vi "ConfigureHW.vi"(8 "error in (no error)":errorcluster, 11 "BME_DG_Base in":refnum<class "BME_DG_Base.lvclass">) -> (0 "error out":errorcluster, 3 "BME_DG_Base out":refnum<class "BME_DG_Base.lvclass">)   [LabVIEW 2009, in "POLARIS BME DG.lvlib" / "BME_DG_Base.lvclass"]
uses:
  BME_DG_Base.lvclass
  BME_DG_Base.lvclass/BME_DG_Base.ctl
  POLARIS BME DG.lvlib
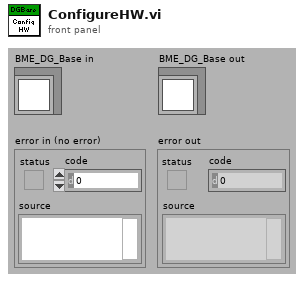
[diagram p1: front panel]
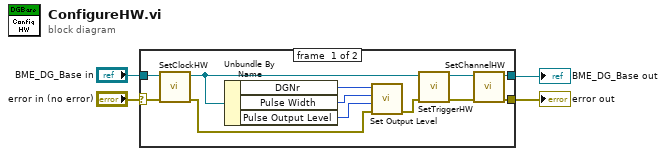
[diagram p0: block diagram]
diagram:
  n1 = case shown="No Error" "error in (no error)" {
    selector: "error in (no error)" -> [w12 w18]
    tunnel: [w11 w18] -> w3
    tunnel: [w14 w17] -> w1
    tunnel: "BME_DG_Base in" -> [w16 w17]
    frame #0 {
      n2 = call-dynamic "SetClockHW.vi"("error in (no error)"=w12, "BME_DG_Base in"=w16) -> ("error out"=w10:errorcluster, "BME_DG_Base out"=w8:refnum<class "BME_DG_Base.lvclass">)  [unwired: 8 in]
      n3 = Unbundle By Name(w8) -> ("DGNr"=w5:i32, "Pulse Width"=w7:u32, "Pulse Output Level"=w6:u32)
      n4 = call "Set Output Level.vi"("error in (no error)"=w10, "Output Level"=w6, "Pulse Width"=w7, "DG Number"=w5) -> ("error out"=w9:errorcluster)  [unwired: 7 in]
      n5 = call-dynamic "SetTriggerHW.vi"("error in (no error)"=w9, "BME_DG_Base in"=w8) -> ("error out"=w13:errorcluster, "BME_DG_Base out"=w15:refnum<class "BME_DG_Base.lvclass">)  [unwired: 8 in]
      n6 = call-dynamic "SetChannelHW.vi"("error in (no error)"=w13, "BME_DG_Base in"=w15) -> ("error out"=w11:errorcluster, "BME_DG_Base out"=w14:refnum<class "BME_DG_Base.lvclass">)  [unwired: 8 in]
    }
    frame #1 {
    }
  }
  "error out" <- w3
  "BME_DG_Base out" <- w1
